vi "DataLogger.vi"(5 "Value":i32, 7 "Operation":T2, 8 "Number of Data Entries":u32=100, 9 "Data Set Name":string="Light", 10 "Filename (no .txt)":string="RedData.dat", 11 "NXT In":T1) -> (3 "NXT Out":T1)   [LabVIEW 2012]
uses:
  RecordDataFileControl.ctl
  <vilib>/NXT/Subs/LVHSConnector.ctl
  <vilib>/NXT/LegoClasses/BrickReference/BrickReference.lvclass
  <vilib>/NXT/Dual Mode Library/Logging/CreateLoggingFile.vi
  <vilib>/NXT/Dual Mode Library/Logging/AddDataPoint.vi
panel:
  # "Proper use is as follows:\n1. Initialize VI with filename and number of values to record\n2. Record each value\n3. Close this VI out"
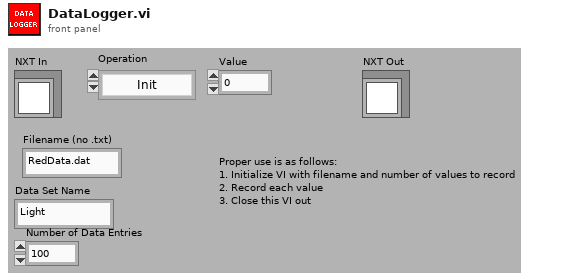
[diagram p1: front panel]
types:
  T1 = typedef "LVHSConnector.ctl" = refnum<class "BrickReference.lvclass">
  T2 = typedef "RecordDataFileControl.ctl" = enum16{"Init", "Delete", "Close", "Record", "Enable", "Disable", "Set Current File"}
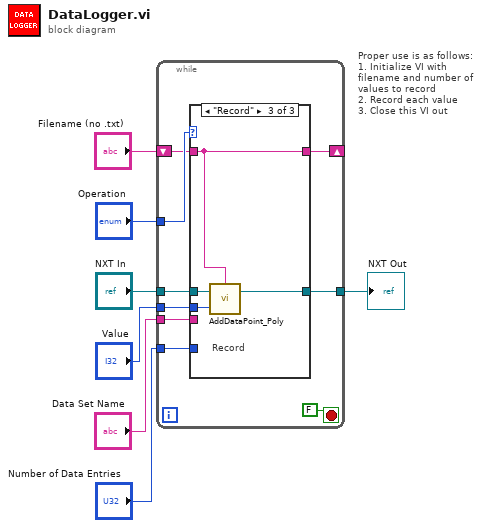
[diagram p0: block diagram]
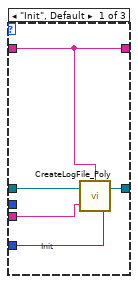
[diagram p2: hidden frame]
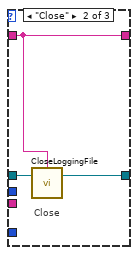
[diagram p3: hidden frame]
diagram:
  # "Proper use is as follows:\n1. Initialize VI with filename and number of values to record\n2. Record each value\n3. Close this VI out"
  n1 = while {
    tunnel: "Operation" -> [w16]
    tunnel: [w14] -> w5
    tunnel: "NXT In" -> [w13]
    shift-right: [w11] -> _
    shift-left: "Filename (no .txt)" -> [w15]
    tunnel: "Data Set Name" -> [w12]
    tunnel: "Number of Data Entries" -> [w10]
    tunnel: "Value" -> [w9]
    stop <- FALSE stop-if-true
    n2 = case shown="\"Record\"" w16 {
      tunnel: w15 -> [w17 w24 w26]
      tunnel: [w21 w22 w27] -> w14
      tunnel: w13 -> [w20 w23 w28]
      tunnel: w12 -> [w19 _ _]
      tunnel: [w17 w24 w26] -> w11
      tunnel: w10 -> [w18 _ _]
      tunnel: w9 -> [_ _ w25]
      frame "Init", Default {
        # "Init"
        n3 = call-poly <vilib>:"CreateLogFile_Poly.vi"("Sensor Name"=w19, "Number of Points"=w18, "NXT"=w20, "Filename"=w17) -> ("NXT"=w21:T1)
      }
      frame "Close" {
        # "Close"
        n4 = call <vilib>:"CloseLoggingFile.vi"("NXT"=w23, "Filename"=w24) -> ("NXT"=w22:T1)  [unwired: 2 in]
      }
      frame "Record" {
        # "Record"
        n5 = call-poly <vilib>:"AddDataPoint_Poly.vi"("Value"=w25, "NXT"=w28, "Filename"=w26) -> ("NXT"=w27:T1)  [unwired: 1 in]
      }
    }
  }
  "NXT Out" <- w5
